vi "GVmotor_move_FP.vi"(8 "error in":errorcluster, 9 "Steps":i32, 10 "wait_ms":u32=100, 11 "VISA in":refnum<visa-resource-name>) -> (0 "error out":errorcluster, 3 "VISA out":refnum<visa-resource-name>)   [LabVIEW 2019]
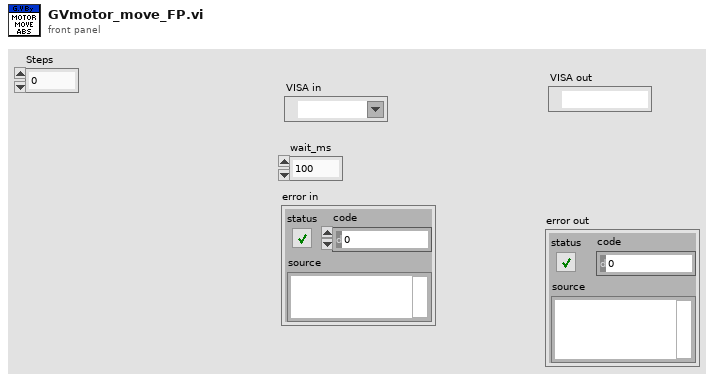
[diagram p1: front panel]
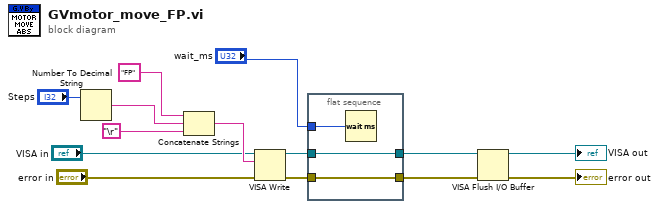
[diagram p0: block diagram]
diagram:
  n1 = Number To Decimal String(number="Steps") -> (decimal integer string=w7:string)  [unwired: 1 in]
  n2 = Concatenate Strings("FP" ("string"), w7, "\r") -> (w14:string)
  n3 = VISA Write(VISA resource name="VISA in", write buffer=w14, error in (no error)="error in") -> (VISA resource name out=w10:refnum<visa-resource-name>, error out=w11:errorcluster)  [unwired: 1 out]
  n4 = flat-sequence {
    tunnel: [w17] -> w5
    tunnel: w11 -> [w17]
    tunnel: [w16] -> w4
    tunnel: w10 -> [w16]
    tunnel: "wait_ms" -> [w15]
    frame #0 {
      n5 = Wait (ms)(milliseconds to wait=w15) -> ()  [unwired: 1 out]
    }
  }
  n6 = VISA Flush I/O Buffer(VISA resource name=w4, error in (no error)=w5) -> (VISA resource name out=→"VISA out":refnum<visa-resource-name>, error out=→"error out":errorcluster)  [unwired: 1 in]
